vi "Print drop FPGA--140614.vi"() -> ()   [LabVIEW 2009]
uses:
  <vilib>/eio/EIONode/EIONode.xnode
  <vilib>/rvi/eio/nirviEIOImplementation/nirviEIOImplementation.xnode
  <vilib>/rvi/eio/common/nirviEmuTemplateMethod_noerrors.vi
  <vilib>/rvi/eio/common/nirviEmuClasses.ctl
  Instance           3 24Saved   Streamlined FPGA .vi
  Instance           4 24Saved   Streamlined FPGA .vi
  Instance           5 24Saved   Streamlined FPGA .vi
  Instance           2 24Saved   Streamlined FPGA .vi
  <vilib>/rvi/DataTransferAndStorage/Container/XNode/niFpgaContainer.xnode
  <vilib>/rvi/interface/RandomDataEmulation/niFpgaRandomDataHandleErrors.vi
  <vilib>/rvi/interface/RandomDataEmulation/nirviRandomDataFPGAFIFO.vi
  <vilib>/rvi/DataTransferAndStorage/Container/Common/niFpgaContainerMethod.ctl
  <vilib>/rvi/DataTransferAndStorage/Container/Common/niFpgaTransferTypeControl.ctl
panel:
  out "N1d":u32
  in  "sort one":bool
  in  "sorting gates":cluster{"[0]":i32, "[1]":i32, "[2]":i32}[](array[cluster])=[{"[0]"=3276800, "[1]"=1000, "[2]"=1}, {"[0]"=3276800, "[1]"=1000, "[2]"=1}, {"[0]"=0, "[1]"=0, "[2]"=0}, {"[0]"=0, "[1]"=0, "[2]"=1}]
  in  "window size":i32
  out "sort!":bool
  in  "Maximum Width":i16
  in  "Maximum Height":i16
  in  "trigger on all":bool
  out "sort pulse":i16
  in  "Baselines":i16[](array[numeric])=[0, 0, 0, 0]
  in  "Sb":i8(ring)=1 items=["PMT1", "PMT2", "PMT3", "PMT4"]
  in  "Sa":i8(ring) items=["PMT1", "PMT2", "PMT3", "PMT4"]
  in  "Sort Case":i8(ring)=1 items=["FP", "Magnitude"]
  out "Full 2":bool
  in  "sort all":bool
  out "Drop counter":u32
  out "sort counter":u32
  in  "PMT to detect drops on":u8
  in  "Minimum Height":i16
  in  "Minimum Width":i16
  in  "Ticks between acquires (Ticks)":u32=200
  in  "Gain 1":i16(slide) scale=-32767.0..32767.0
  in  "Gain 2":i16(slide) scale=-32767.0..32767.0
  in  "Gain 3":i16(slide) scale=-32767.0..32767.0
  in  "Gain 4":i16(slide) scale=-32767.0..32767.0
  in  "amplitude":i16
  in  "1/Frequency \n(ticks)":u32
  in  "Burst \nCycles":i32
  in  "delay [us]":u32=20 min=1 max=8000
  # "Acquisition and Detection"
  # "FP and Sorting Parameters"
  # "Sorting Pulse\nGenerator"
  # "Events"
  # "PMT Controls"
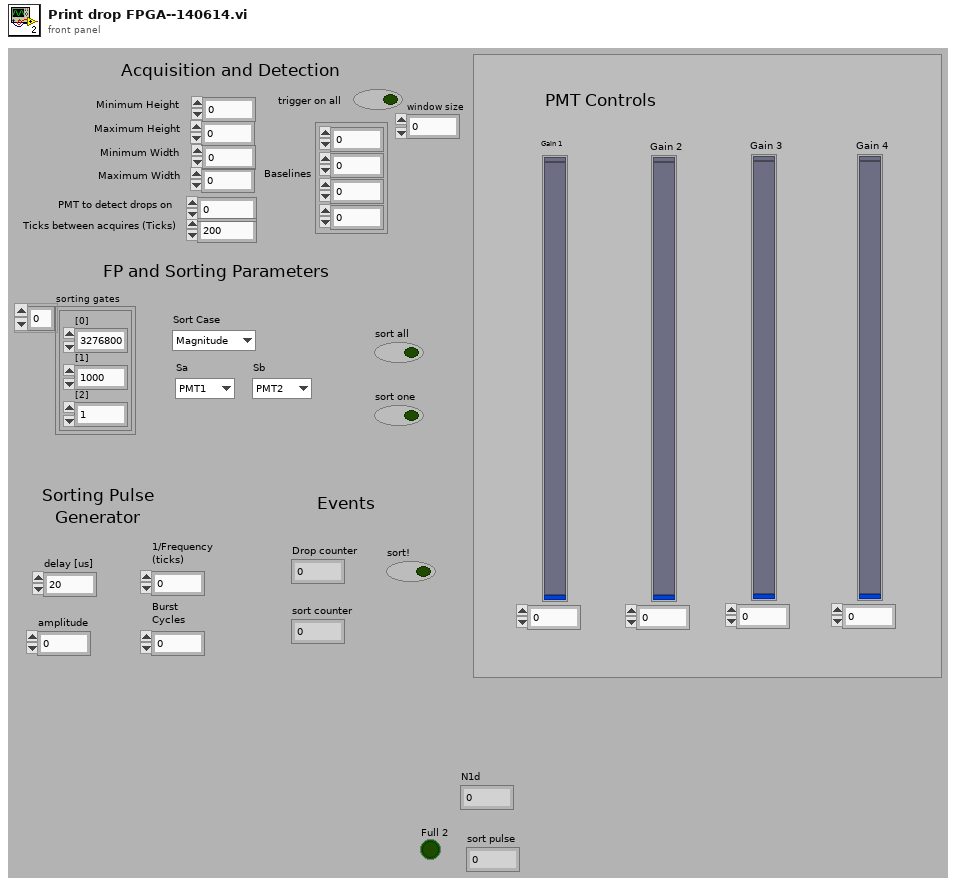
[diagram p1: front panel]
types:
  T1 = typedef "nirviEmuClasses.ctl" = enum16{"IO Read", "IO Write", "Method", "Property Read", "Property Write"}
  T2 = typedef "niFpgaContainerMethod.ctl" = enum16{"Write", "Read", "Clear", "Get Number of Elements to Write", "Get Number of Elements to Read", "Enable", "Disable", "Flush and Disable", "Get Stream State"}
  T3 = typedef "niFpgaTransferTypeControl.ctl" = enum16{"Target-Scoped", "Host to Target - DMA", "Target to Host - DMA", "Peer to Peer Reader", "Peer to Peer Writer", "Bidirectional"}
  T4 = cluster{bool, "max":i16[], "sum":i32[], "time inside":i32, "time outside":i32, "timeoutside-1":i32}
  T5 = cluster{"maxes":i16[], "sums":i32[], "time inside":i32, "time outside":i32}
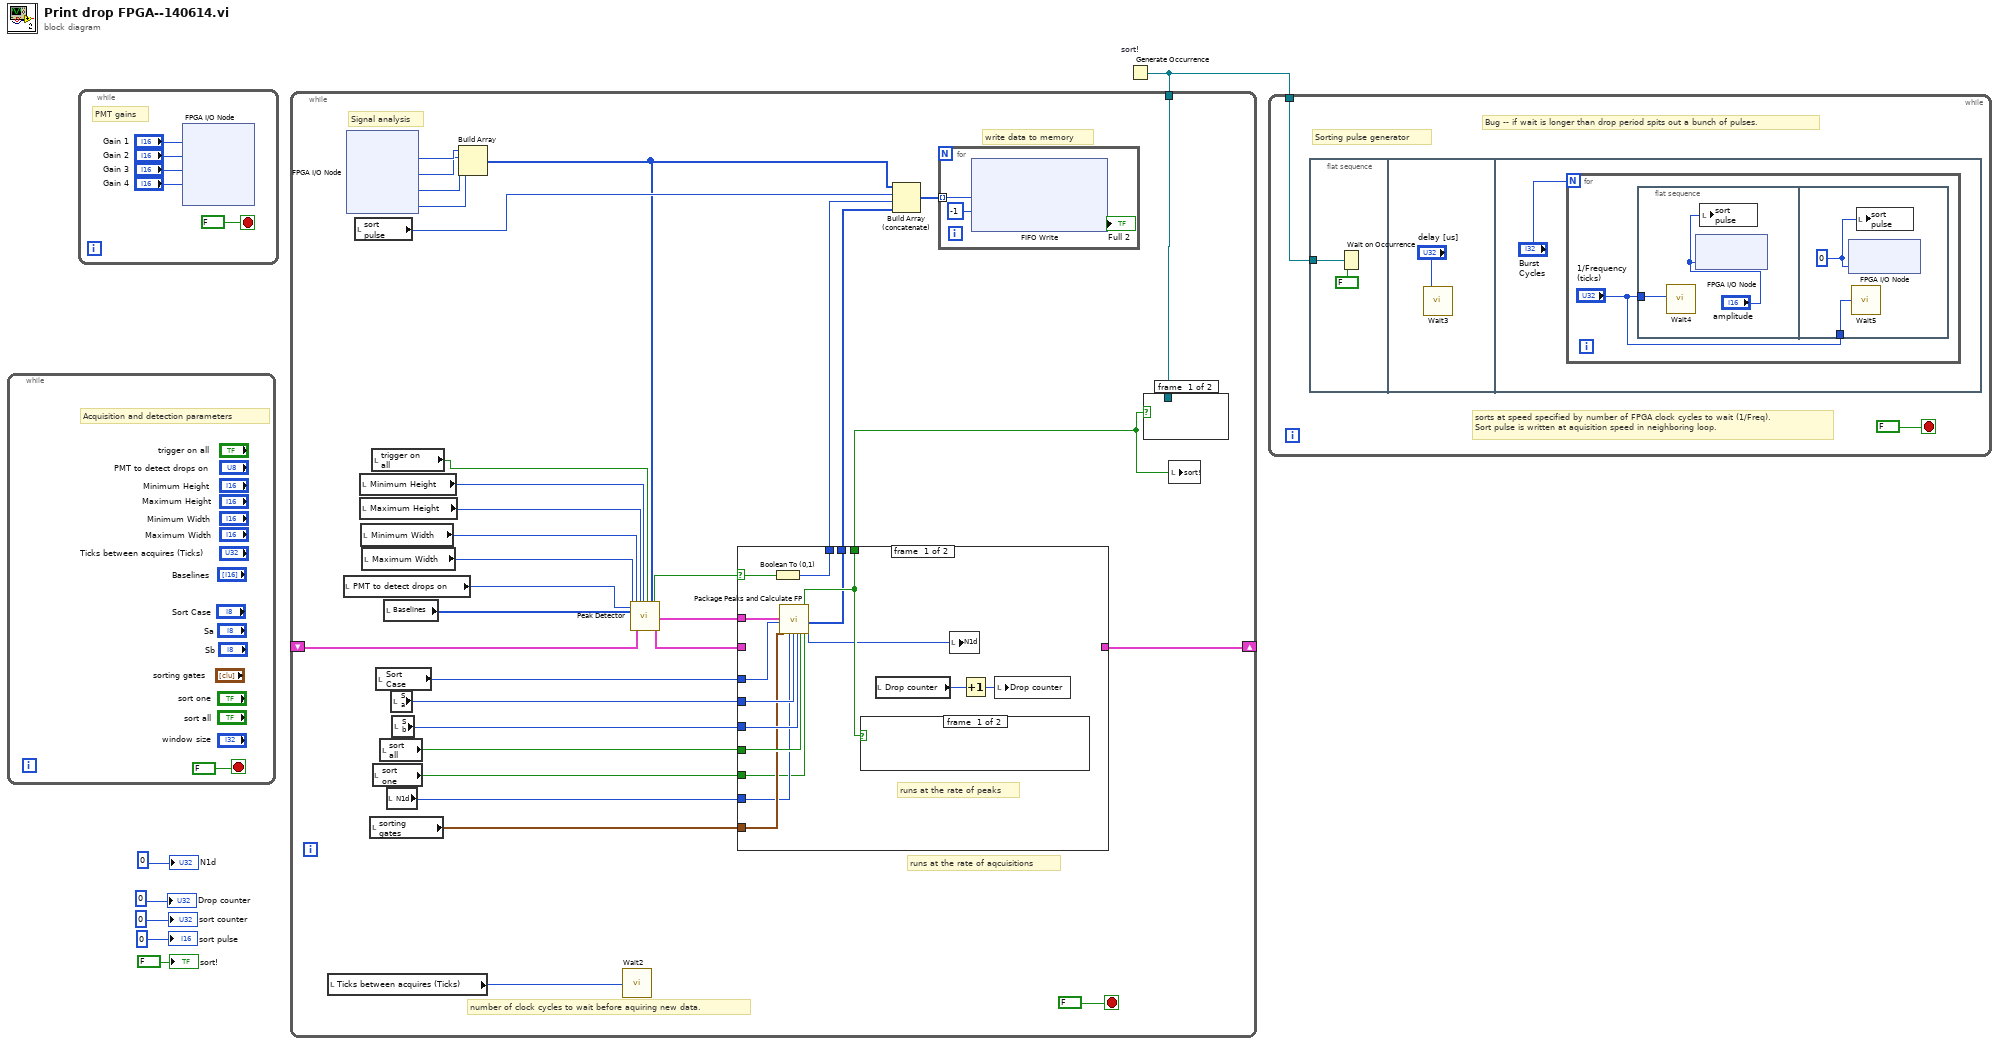
[diagram p0: block diagram]
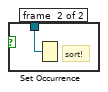
[diagram p2: hidden frame]
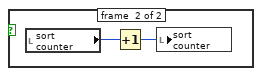
[diagram p3: hidden frame]
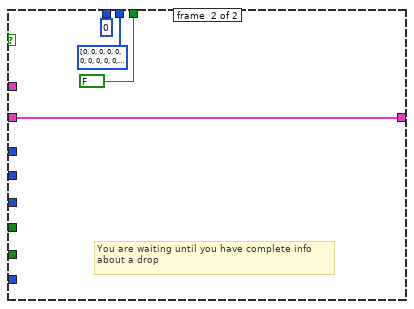
[diagram p4: hidden frame]
diagram:
  n1 = while {
    stop <- FALSE stop-if-true
    # "Acquisition and detection parameters"
  }
  n2 = while {
    stop <- FALSE stop-if-true
    # "PMT gains"
    n3 = xnode "FPGA I/O Node"("AO0"="Gain 1", "AO1"="Gain 2", "AO2"="Gain 3", "AO3"="Gain 4") -> ()  [unwired: 4 in, 4 out]
  }
  n4 = Generate Occurrence "sort!"() -> (w6:refnum<k4>)
  n5 = while {
    shift-right: [w87] -> _
    shift-left: _ -> [w75]
    tunnel: w6 -> [w74]
    stop <- FALSE stop-if-true
    # "runs at the rate of aqcuisitions"
    # "number of clock cycles to wait before aquiring new data."
    # "Signal analysis"
    # "write data to memory"
    n6 = local read "Ticks between acquires (Ticks)"() -> (w82:u32)
    n7 = local read "PMT to detect drops on"() -> (w66:u8)
    n8 = xnode "FPGA I/O Node"() -> ("AI0"=w86:i16, "AI1"=w85:i16, "AI2"=w84:i16, "AI3"=w83:i16)  [unwired: 4 in, 4 out]
    n9 = local read "sort pulse"() -> (w73:i16)
    n10 = local read "Minimum Height"() -> (w70:i16)
    n11 = local read "Maximum Height"() -> (w69:i16)
    n12 = local read "Minimum Width"() -> (w68:i16)
    n13 = local read "Maximum Width"() -> (w67:i16)
    n14 = local read "sorting gates"() -> (w57:cluster{"[0]":i32, "[1]":i32, "[2]":i32}[])
    n15 = local read "trigger on all"() -> (w62:bool)
    n16 = local read "sort one"() -> (w59:bool)
    n17 = local read "Sort Case"() -> (w81:i8)
    n18 = local read "sort all"() -> (w61:bool)
    n19 = local read "Baselines"() -> (w65:i16[])
    n20 = local read "N1d"() -> (w58:u32)
    n21 = local read "Sa"() -> (w80:i8)
    n22 = local read "Sb"() -> (w79:i8)
    n23 = Build Array(w86, w85, w84, w83) -> (w63:i16[])
    n24 = call "Wait2"("Count(Ticks)"=w82) -> ()  [unwired: 1 out]
    n25 = call "Peak Detector.vi"("Maximum Width"=w67, "PMT to trigger on (0,1,2,3)"=w66, "Baselines"=w65, "Minimum Width"=w68, "shifts in"=w75, "Maximum Height"=w69, "Minimum Height"=w70, "trigger on all"=w62, "s1,s2,s3,s4"=w63) -> ("peak complete?"=w78:bool, "shifts out"=w76:T4, "peaks data"=w77:T5)  [unwired: 16 in]
    n26 = case shown="True" w78 {
      selector: w78 -> [w202 _]
      tunnel: [_ w213] -> w87
      tunnel: [w200 FALSE ("sort!")] -> w60
      tunnel: w81 -> [w198 _]
      tunnel: w80 -> [w206 _]
      tunnel: w79 -> [w205 _]
      tunnel: w61 -> [w204 _]
      tunnel: w76 -> [_ w213]
      tunnel: w77 -> [w203 _]
      tunnel: [w201 i16 0] -> w71
      tunnel: [w199 i32[] [0, 0, 0, 0, 0, 0, 0, 0, 0, 0, 0, 0] ("M1,M2,M3,M4,S1,S2,S3,S4,Tin,Tout,FP")] -> w64
      tunnel: w57 -> [w197 _]
      tunnel: w59 -> [w195 _]
      tunnel: w58 -> [w196 _]
      frame #0 {
        # "runs at the rate of peaks"
        n27 = Boolean To (0,1)(Boolean=w202) -> (0, 1=w201:i16)
        n28 = call "Package Peaks and Calculate FP.vi"("peaks data"=w203, "Sort Case"=w198, "Array 2"=w197, "N1d in"=w196, "Sa"=w206, "Sb"=w205, "sort all"=w204, "sort one"=w195) -> ("sort!"=w200:bool, "M1,M2,M3,M4,S1,S2,S3,S4,Tin,Tout,FP,Sort?"=w199:i32[], "N1d out"=w194:u32)  [unwired: 17 in]
        n29 = case shown="True" w200 {
          frame #0 {
          }
          frame #1 {
            n30 = local read "sort counter"() -> (w210:u32)
            n31 = Increment(x=w210) -> (x+1=w209:u32)
            n32 = local write "sort counter"(w209) -> ()
          }
        }
        n33 = local read "Drop counter"() -> (w208:u32)
        n34 = local write "N1d"(w194) -> ()
        n35 = Increment(x=w208) -> (x+1=w207:u32)
        n36 = local write "Drop counter"(w207) -> ()
      }
      frame #1 {
        # "You are waiting until you have complete info about a drop"
      }
    }
    n37 = Build Array (concatenate)(w63, w73, w71, w64) -> (w72:i32[])
    n38 = for {
      tunnel: w72 -> [w92] mode=indexing
      n39 = xnode ("FIFO Write")("Element"=w92, "Timeout"=-1) -> ("Timed Out?"=→"Full 2":bool)  [unwired: 1 in, 1 out]
    }
    n40 = case shown="True" w60 {
      tunnel: w74 -> [_ w89]
      frame #0 {
      }
      frame #1 {
        # "sort!"
        n41 = Set Occurrence(w89) -> ()
      }
    }
    n42 = local write "sort!"(w60) -> ()
  }
  n43 = while {
    tunnel: w6 -> [w215]
    stop <- FALSE stop-if-true
    # "Bug -- if wait is longer than drop period spits out a bunch of pulses."
    # "sorts at speed specified by number of FPGA clock cycles to wait (1/Freq).\nSort pulse is written at aquisition speed in neighboring loop."
    # "Sorting pulse generator"
    n44 = flat-sequence {
      tunnel: w215 -> [w217]
      frame #0 {
        n45 = Wait on Occurrence(1:FALSE ("ignore previous (T)"), 2:w217) -> ()  [unwired: 1 in, 1 out]
      }
      frame #1 {
        n46 = call "Wait3"("Count(uSec)"="delay [us]") -> ()  [unwired: 1 out]
      }
      frame #2 {
        n47 = for {
          N: "Burst \nCycles" -> [_]
          n48 = flat-sequence {
            tunnel: "1/Frequency \n(ticks)" -> [w223]
            tunnel: "1/Frequency \n(ticks)" -> [w236]
            frame #0 {
              n49 = call "Wait4"("Count(Ticks)"=w223) -> ()  [unwired: 1 out]
              n50 = xnode "FPGA I/O Node"("AO4"="amplitude") -> ()  [unwired: 1 in, 1 out]
              n51 = local write "sort pulse"("amplitude") -> ()
            }
            frame #1 {
              w235 = i16 0 ("sort pulse")
              n52 = xnode "FPGA I/O Node"("AO4"=w235) -> ()  [unwired: 1 in, 1 out]
              n53 = call "Wait5"("Count(Ticks)"=w236) -> ()  [unwired: 1 out]
              n54 = local write "sort pulse"(w235) -> ()
            }
          }
        }
      }
    }
  }
  "sort counter" <- u32 0 ("event counter")
  "Drop counter" <- u32 0 ("Drop counter")
  "sort pulse" <- i16 0 ("event counter")
  "sort!" <- FALSE ("sort!")
  "N1d" <- u32 0 ("Drop counter")
